vi "Refname to String (Motors).vi"(1 "Enum":T1) -> (0 "String":string)   [LabVIEW 2016]
uses:
  Motors.ctl
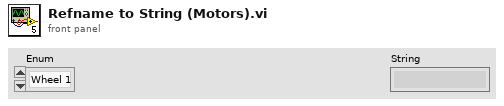
[diagram p1: front panel]
types:
  T1 = typedef "Motors.ctl" = enum16{"Wheel 1", "Swerve 1"}
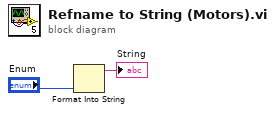
[diagram p0: block diagram]
diagram:
  n1 = Format Into String("Enum") -> (resulting string=→"String":string)  [unwired: 3 in, 1 out]
